vi "ReplacementArray1.vi"(3 "Value for replace":dbl, 4 "Starting Index":i32, 5 "Replaced Array IN":dbl[](array[numeric])) -> (1 "Finishing Index (n+1)":i32, 2 "Replaced Array OUT":dbl[](array[numeric]))   [LabVIEW 2013]
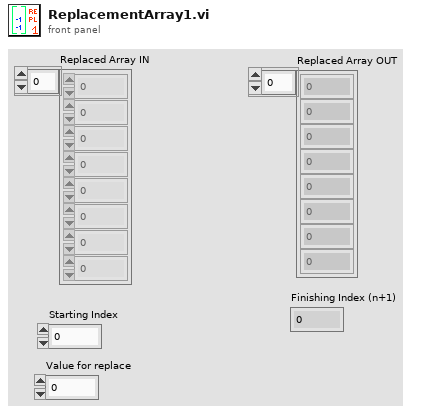
[diagram p1: front panel]
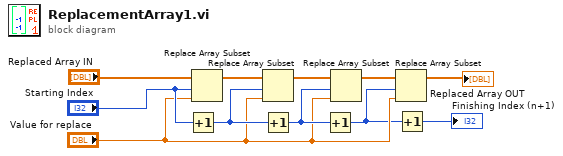
[diagram p0: block diagram]
diagram:
  n1 = Increment(x="Starting Index") -> (x+1=w8:i32)
  n2 = Replace Array Subset(array="Replaced Array IN", new element="Value for replace", index="Starting Index") -> (w9:dbl[])
  n3 = Replace Array Subset(array=w9, new element="Value for replace", index=w8) -> (w7:dbl[])
  n4 = Increment(x=w8) -> (x+1=w6:i32)
  n5 = Increment(x=w6) -> (x+1=w3:i32)
  n6 = Replace Array Subset(array=w7, new element="Value for replace", index=w6) -> (w5:dbl[])
  n7 = Replace Array Subset(array=w5, new element="Value for replace", index=w3) -> (→"Replaced Array OUT":dbl[])
  n8 = Increment(x=w3) -> (x+1=→"Finishing Index (n+1)":i32)
